vi "DigitalIn_read.vi"(8 "error in (no error)":errorcluster, 11 "DigitalIn in":refnum<class "DigitalIn.lvclass">) -> (0 "error out":errorcluster, 2 "Value":bool, 3 "DigitalIn out":refnum<class "DigitalIn.lvclass">)   [LabVIEW 2011, in "mbed_LVLibrary.lvlib" / "DigitalIn.lvclass"]
uses:
  DigitalIn.lvclass
  DigitalIn.lvclass/DigitalIn.ctl
  Transport Mechanisms/mbed/mbed.lvclass
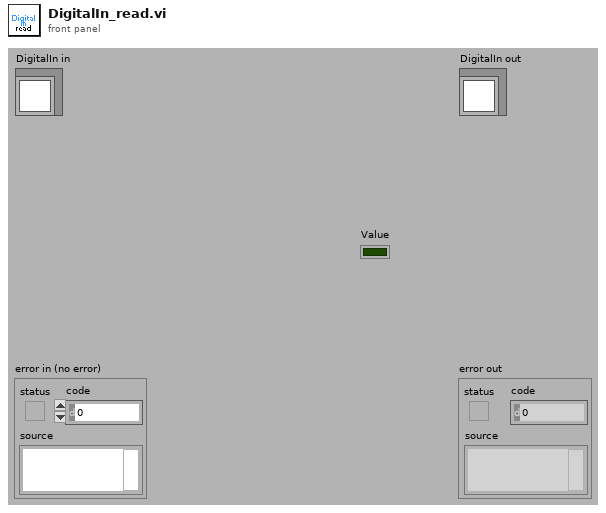
[diagram p1: front panel]
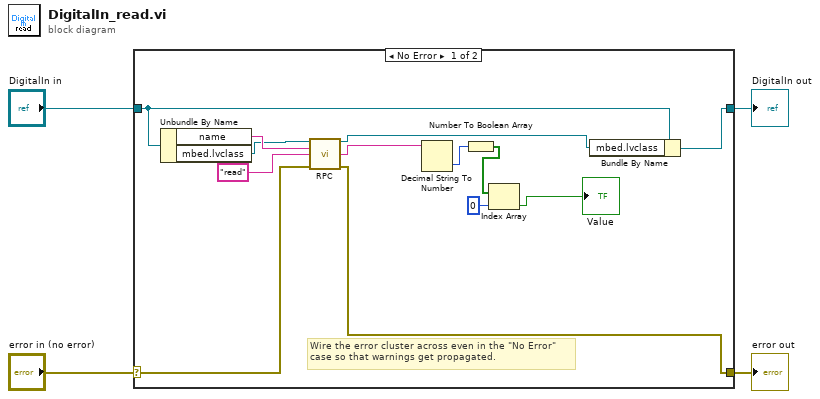
[diagram p0: block diagram]
diagram:
  n1 = case shown="No Error" "error in (no error)" {
    selector: "error in (no error)" -> [w6 w19]
    tunnel: [w5 w19] -> w3
    tunnel: [w8 w18] -> w1
    tunnel: "DigitalIn in" -> [w9 w18]
    frame No Error {
      # "Wire the error cluster across even in the \"No Error\"\ncase so that warnings get propagated."
      n2 = Unbundle By Name(w9) -> ("name"=w13:string, "mbed.lvclass"=w12:refnum<class "mbed.lvclass">)
      n3 = call-dynamic "RPC.vi"("mbed in"=w12, "Name"=w13, "method"="read", "error in (no error)"=w6) -> ("mbed out"=w7:refnum<class "mbed.lvclass">, "RPC Result"=w10:string, "error out"=w5:errorcluster)  [unwired: 9 in]
      n4 = Decimal String To Number(string=w10) -> (number=w15:i32)  [unwired: 2 in, 1 out]
      n5 = Number To Boolean Array(number=w15) -> (Boolean array=w17:bool[])
      n6 = Index Array(array=w17, index=0) -> (element=→"Value":bool)
      n7 = Bundle By Name(cluster=w9, "mbed.lvclass"=w7) -> (w8:refnum<class "DigitalIn.lvclass">)
    }
    frame Error {
    }
  }
  "error out" <- w3
  "DigitalIn out" <- w1
